vi "OAT Compensate Even Angle Signal (Even Angle Ref, N Channels).vi"(0 "even-angle signals":cluster{"r0":dbl, "dr":dbl, "Y":dbl[]}[](array[cluster]) {"r0" format="%.2p"; "dr" format="%.2p"; "Y" format="%.2f"}, 2 "reset? (F)":bool, 5 "even-angle references":cluster{"r0":dbl, "dr":dbl, "Y":dbl[]}[](array[cluster]) {"r0" format="%.2p"; "dr" format="%.2p"; "Y" format="%.2f"}, 7 "even-angle position info":T1, 9 "speed profile":T2 {"speed [RPM]" format="%.2f"; "time [s]" format="%.2f"}, 11 "error in (no error)":errorcluster) -> (4 "compensated even-angle signals":cluster{"r0":dbl, "dr":dbl, "Y":dbl[]}[](array[cluster]) {"r0" format="%.2p"; "dr" format="%.2p"; "Y" format="%.2f"}, 6 "actual even-angle references":cluster{"r0":dbl, "dr":dbl, "Y":dbl[]}[](array[cluster]) {"r0" format="%.2p"; "dr" format="%.2p"; "Y" format="%.2f"}, 8 "even-angle position info out":T1, 15 "error out":errorcluster)   [LabVIEW 2017, in "SoundVib_RefDataProcess.lvlib"]
doc: "Compensates an even-angle signal. You can use the <B>compensated even-angle signal</B> output to display unfiltered orbit and timebase plots with the runout pattern removed. Wire data to the <B>even-angle signal</B> input to determine the polymorphic instance to use or manually select the instance."
uses:
  <vilib>/addons/Sound and Vibration/Order Analysis/Referece Data Processing/SoundVib_RefDataProcess.lvlib
  <vilib>/addons/Sound and Vibration/Order Analysis/Misc/OAT Position Info.ctl
  <vilib>/addons/Sound and Vibration/Order Analysis/Tach Process/SubVIs/speed profile.ctl
  <vilib>/addons/Sound and Vibration/Order Analysis/Resample Order Tracking/SoundVib_Resampling.lvlib
  <vilib>/addons/Sound and Vibration/Order Analysis/Tach Process/SoundVib_TachProcess.lvlib
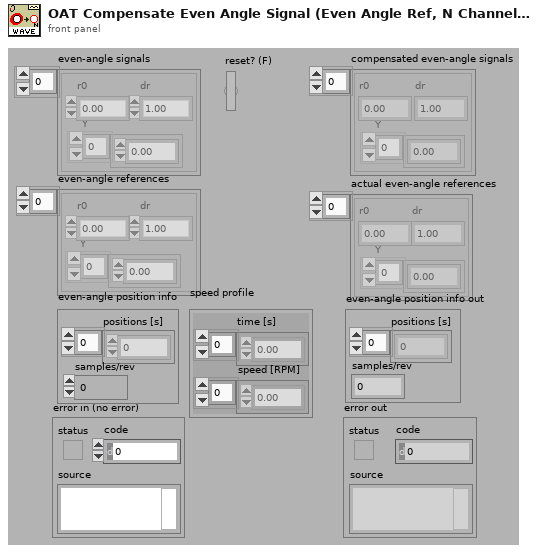
[diagram p1: front panel]
types:
  T1 = typedef "OAT Position Info.ctl" = cluster{"positions [s]":dbl[], "samples/rev":dbl}
  T2 = typedef "SoundVib_TachProcess.lvlib/speed profile.ctl" = cluster{"time [s]":dbl[], "speed [RPM]":dbl[]}
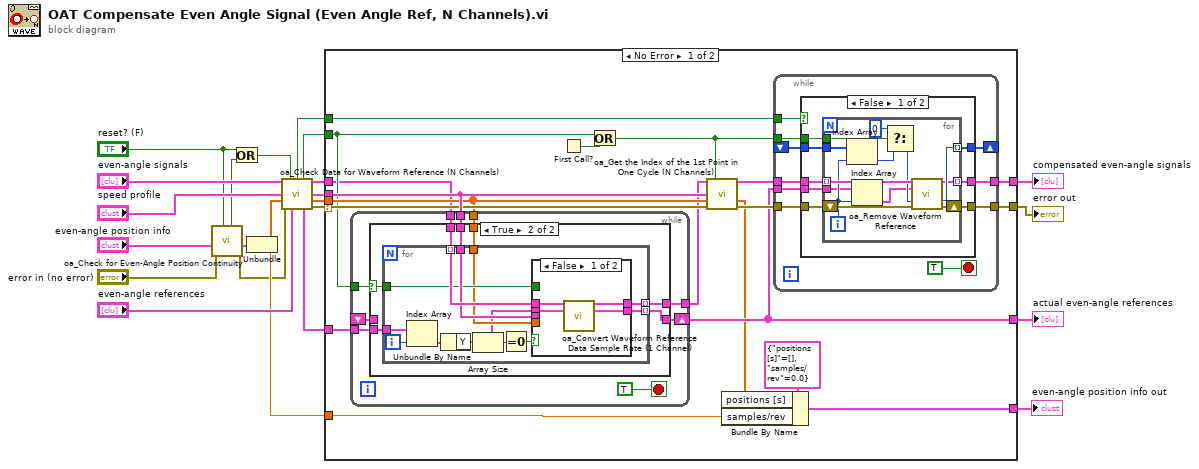
[diagram p0: block diagram]
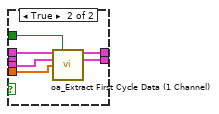
[diagram p3: hidden frame]
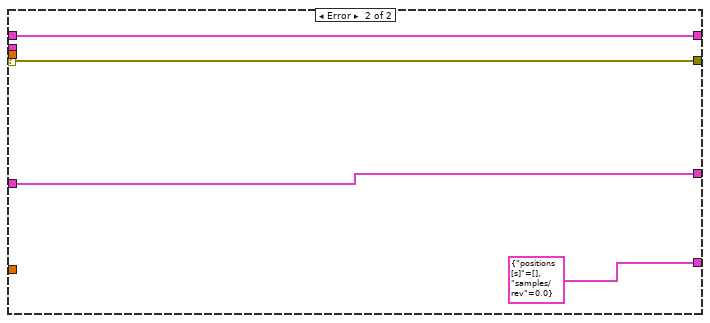
[diagram p5: hidden frame]
diagram:
  n1 = call <vilib>:"oa_Check for Even-Angle Position Continuity.vi"("reset in"="reset? (F)", "error in (no error)"="error in (no error)", "even-angle position info"="even-angle position info") -> ("error out"=w4:errorcluster, "even-angle position info dup"=w6:T1, "position not continuous"=w2:bool)  [unwired: 6 in]
  n2 = Or(x="reset? (F)", y=w2) -> (x .or. y?=w1:bool)
  n3 = Unbundle(w6) -> ("positions [s]"=w15:dbl[], "samples/rev"=w9:dbl)
  n4 = call <vilib>:"oa_Check Data for Waveform Reference (N Channels).vi"("resampled signal"="even-angle signals", "reset? (True)"=w1, "speed profile"="speed profile", "interpolated pulse positions"=w15, "error in (no error)"=w4, "even angle references in"="even-angle references") -> ("empty signal?"=w11:bool, "reset"=w13:bool, "resampled data out"=w22:cluster{"r0":dbl, "dr":dbl, "Y":dbl[]}[], "speed profile out"=w21:T2, "interpolated pulse positions out"=w20:dbl[], "even angle references out"=w12:cluster{"r0":dbl, "dr":dbl, "Y":dbl[]}[], "error out"=w23:errorcluster)  [unwired: 2 in, 1 out]
  n5 = case shown="No Error" w23 {
    selector: w23 -> [w41 w120]
    tunnel: w22 -> [w30 w119]
    tunnel: w21 -> [w42 _]
    tunnel: w20 -> [w37 _]
    tunnel: [w39 w119] -> w17
    tunnel: [w31 w118] -> w18
    tunnel: [w38 w120] -> w16
    tunnel: w13 -> [w35 _]
    tunnel: w12 -> [w33 w118]
    tunnel: w11 -> [w32 _]
    tunnel: w9 -> [w25 _]
    tunnel: [w24 T1 {"positions [s]"=[], "samples/rev"=0.0} ("even angle position info")] -> w8
    frame No Error {
      n6 = while {
        tunnel: w30 -> [w51]
        tunnel: w42 -> [w50]
        tunnel: w35 -> [w45]
        tunnel: [w49] -> w28
        tunnel: w37 -> [w48]
        tunnel: w33 -> [w47]
        shift-right: [w44] -> w31
        shift-left: _ -> [w43]
        stop <- TRUE stop-if-true
        n7 = case shown="True" w45 {
          selector: w45 -> [_ w55]
          tunnel: w51 -> [w52 w60]
          tunnel: w50 -> [_ w59]
          tunnel: [w53 w54] -> w44
          tunnel: [w52 w58] -> w49
          tunnel: w48 -> [_ w57]
          tunnel: w47 -> [_ w56]
          tunnel: w43 -> [w53 _]
          frame False {
          }
          frame True {
            n8 = for {
              tunnel: w60 -> [w72] mode=indexing
              tunnel: w59 -> [w71]
              tunnel: w55 -> [w70]
              tunnel: [w69] -> w58 mode=indexing
              tunnel: w57 -> [w68]
              tunnel: w56 -> [w64]
              tunnel: [w61] -> w54 mode=indexing
              i -> [w63]
              n9 = Index Array(array=w64, index=w63) -> (element=w62:cluster{"r0":dbl, "dr":dbl, "Y":dbl[]})
              n10 = Unbundle By Name(w62) -> ("Y"=w67:dbl[])
              n11 = Array Size(array=w67) -> (size(s)=w66:i32)
              n12 = Equal To 0?(x=w66) -> (x = 0?=w65:bool)
              n13 = case shown="False" w65 {
                tunnel: w62 -> [w75 _]
                tunnel: [w73 w79] -> w61
                tunnel: w72 -> [w76 w82]
                tunnel: w70 -> [_ w81]
                tunnel: w71 -> [_ w78]
                tunnel: [w74 w80] -> w69
                tunnel: w68 -> [_ w77]
                frame False {
                  n14 = call <vilib>:"oa_Convert Waveform Reference Data Sample Rate (1 Channel).vi"("resampled signal"=w76, "baseline in"=w75) -> ("resampled signal dup"=w74:cluster{"r0":dbl, "dr":dbl, "Y":dbl[]}, "baseline in out"=w73:cluster{"r0":dbl, "dr":dbl, "Y":dbl[]})  [unwired: 11 in, 1 out]
                }
                frame True {
                  n15 = call <vilib>:"oa_Extract First Cycle Data (1 Channel).vi"("resampled signal"=w82, "reset? (True)"=w81, "speed profile"=w78, "interpolated pulse positions"=w77) -> ("resampled signal out"=w80:cluster{"r0":dbl, "dr":dbl, "Y":dbl[]}, "waveform reference data"=w79:cluster{"r0":dbl, "dr":dbl, "Y":dbl[]})  [unwired: 9 in, 1 out]
                }
              }
            }
          }
        }
      }
      n16 = First Call?() -> (First Call?: T/F=w34:bool)
      n17 = Or(x=w35, y=w34) -> (x .or. y?=w36:bool)
      n18 = call <vilib>:"oa_Get the Index of the 1st Point in One Cycle (N Channels).vi"("resampled signal"=w28, "reset? (True)"=w36, "speed profile"=w42, "interpolated pulse positions"=w37, "error in (no error)"=w41) -> ("resampled signal out"=w29:cluster{"r0":dbl, "dr":dbl, "Y":dbl[]}[], "interpolated pulse positions out"=w26:dbl[], "error out"=w40:errorcluster)  [unwired: 8 in]
      n19 = Bundle By Name(cluster=T1 {"positions [s]"=[], "samples/rev"=0.0} ("even angle position info"), "positions [s]"=w26, "samples/rev"=w25) -> (w24:T1)
      n20 = while {
        tunnel: w40 -> [w92]
        tunnel: [w91] -> w38
        tunnel: w31 -> [w89]
        shift-right: [w88] -> _
        shift-left: _ -> [w84]
        tunnel: w36 -> [w85]
        tunnel: w29 -> [w86]
        tunnel: [w87] -> w39
        tunnel: w32 -> [w83]
        stop <- TRUE stop-if-true
        n21 = case shown="False" w83 {
          tunnel: w92 -> [w100 w114]
          tunnel: [w99 w114] -> w91
          tunnel: w89 -> [w98 _]
          tunnel: [w97 w116] -> w88
          tunnel: [w96 w115] -> w87
          tunnel: w86 -> [w95 w115]
          tunnel: w85 -> [w94 _]
          tunnel: w84 -> [w93 w116]
          frame False {
            n22 = for {
              tunnel: w98 -> [w102]
              tunnel: [w111] -> w97 mode=indexing
              tunnel: [w110] -> w96 mode=indexing
              tunnel: w95 -> [w109] mode=indexing
              shift-right: [w112] -> w99
              shift-left: w100 -> [w113]
              tunnel: w94 -> [w107]
              tunnel: w93 -> [w106]
              i -> [w103]
              n23 = Index Array(array=w106, index=w103) -> (element=w105:i32)
              n24 = Index Array(array=w102, index=w103) -> (element=w101:cluster{"r0":dbl, "dr":dbl, "Y":dbl[]})
              n25 = Select(t=0, s=w107, f=w105) -> (s? t:f=w104:i32)
              n26 = call <vilib>:"oa_Remove Waveform Reference.vi"("resampled signal"=w109, "baseline in"=w101, "last index"=w104, "error out in"=w113) -> ("compensated signal"=w110:cluster{"r0":dbl, "dr":dbl, "Y":dbl[]}, "last index out"=w111:i32, "error out"=w112:errorcluster)  [unwired: 9 in]
            }
          }
          frame True {
          }
        }
      }
    }
    frame Error {
    }
  }
  "error out" <- w16
  "compensated even-angle signals" <- w17
  "actual even-angle references" <- w18
  "even-angle position info out" <- w8
